vi "Read Time.vi"(8 "error in (no error)":errorcluster, 11 "FormulaG API in":refnum<class "FormulaG API.lvclass">) -> (0 "error out":errorcluster, 1 "Last Lap":dbl format="%<%M:%S%3u>t", 2 "Current Lap":dbl format="%<%M:%S%3u>t", 3 "FormulaG API out":refnum<class "FormulaG API.lvclass">)   [LabVIEW 2020, in "FormulaG.lvlib" / "FormulaG API.lvclass"]
uses:
  FormulaG API.lvclass
  Command.ctl
  FormulaG API.lvclass/FormulaG API.ctl
  <vilib>/IlluminatedG/lv-stream/stream/Stream.lvclass/Stream.ctl
  <vilib>/IlluminatedG/lv-stream/stream/Dispatch Sniffer Data.vi
  <vilib>/IlluminatedG/lv-stream/stream/Prepared.vi
  <vilib>/IlluminatedG/lv-stream/Endpoint/Cast Sniffer Callback.vi
  <vilib>/IlluminatedG/IG WebSocket Stream/Stream-Websocket/WebsocketStream/WebsocketStream.lvclass
  C:/Program Files (x86)/National Instruments/LabVIEW 2020/vi.lib/IlluminatedG/lv-stream/stream/Stream.lvclass
  <vilib>/Utility/error.llb/Error Cluster From Error Code.vi
  <vilib>/IlluminatedG/lv-stream/stream/Stream.lvclass
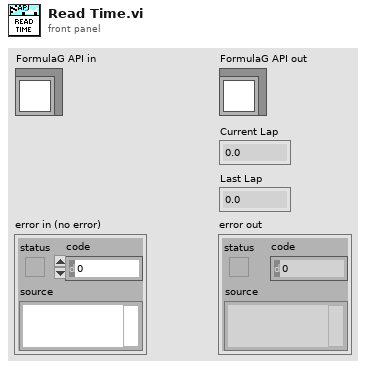
[diagram p1: front panel]
types:
  T1 = enum16{"big-endian, network order", "native, host order", "little-endian"}
  T2 = typedef "FormulaG.lvlib/FormulaG API.lvclass/Command.ctl" = enum8{"None", "Reset Car", "Request Ranges", "Control Car", "Request Info", "Set Options", "Set Camera", "Set Pause", "Request Time"}
  T3 = cluster{"U8":u8, "Current Lap mS":i64, "Last Lap mS":i64}
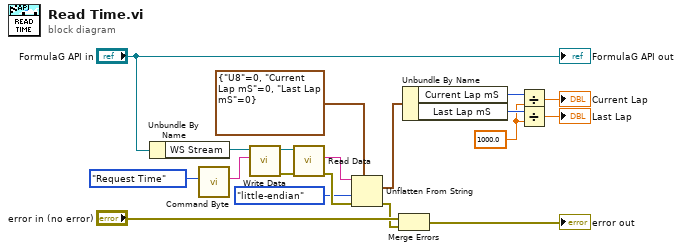
[diagram p0: block diagram]
diagram:
  w5 = 1000.0
  n1 = Unbundle By Name("FormulaG API in") -> ("WS Stream"=w17:refnum<class "WebsocketStream.lvclass">)
  n2 = call "Command Byte.vi"("Command"=Command."Request Time") -> ("Command Byte"=w15:string)  [unwired: 10 in]
  n3 = call <vilib>:"Write Data.vi"("Data"=w15, "Stream in"=w17) -> ("error out"=w13:errorcluster, "Stream out"=w14:refnum<class "WebsocketStream.lvclass">)  [unwired: 8 in]
  n4 = call <vilib>:"Read Data.vi"("error in (no error)"=w13, "Stream in"=w14) -> ("error out"=w12:errorcluster, "Data"=w10:string)  [unwired: 7 in, 1 out]
  n5 = Unflatten From String(type=T3 {"U8"=0, "Current Lap mS"=0, "Last Lap mS"=0}, binary string=w10, byte order (0:big-endian, network order)=T1."little-endian", error in (no error)=w12) -> (value=w8:T3, error out=w1:errorcluster)  [unwired: 1 in, 1 out]
  n6 = Merge Errors("error in (no error)", w1) -> (→"error out":errorcluster)
  n7 = Unbundle By Name(w8) -> ("Current Lap mS"=w7:i64, "Last Lap mS"=w6:i64)
  n8 = Divide(x=w7, y=w5) -> (x/y=→"Current Lap":dbl)
  n9 = Divide(x=w6, y=w5) -> (x/y=→"Last Lap":dbl)
  "FormulaG API out" <- "FormulaG API in"
